vi "ToString.vi"(8 "error in (no error)":errorcluster, 11 "Fact in":refnum<class "Fact.lvclass">) -> (0 "error out":errorcluster, 2 "String":string, 3 "Fact out":refnum<class "Fact.lvclass">)   [LabVIEW 2019, in "Fact.lvclass"]
doc: "Returns the string representation for this object."
uses:
  Fact.lvclass
  Fact.lvclass/Fact.ctl
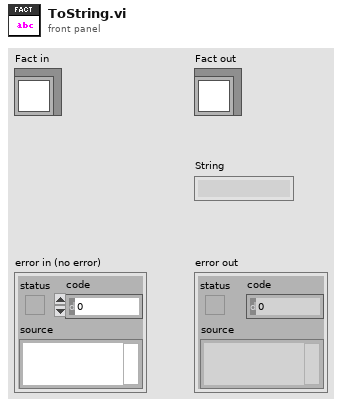
[diagram p1: front panel]
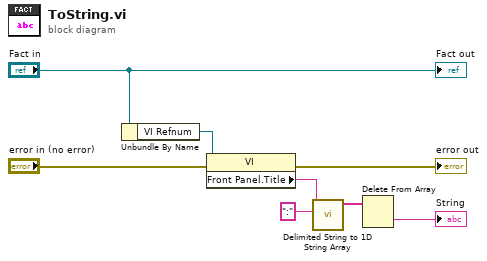
[diagram p0: block diagram]
diagram:
  n1 = Unbundle By Name("Fact in") -> ("VI Refnum"=w5:refnum<vi>)
  n2 = property class="VI"(reference=w5, error in="error in (no error)") -> (error out=→"error out":errorcluster, "Front Panel.Title"=w3:string)  [unwired: 1 out]
  n3 = call <vilib>:"Delimited String to 1D String Array.vi"("delimiter"=":", "delimited string"=w3) -> ("string array"=w2:string[])  [unwired: 9 in]
  n4 = Delete From Array(array=w2) -> (deleted portion=→"String":string)  [unwired: 2 in, 1 out]
  "Fact out" <- "Fact in"
